vi "Mediciones4.vi"(0 "OK Button":bool, 1 "Alto":dbl, 2 "Ancho":dbl) -> ()   [LabVIEW 2017]
panel:
  out "Array":dbl[](array[numeric])
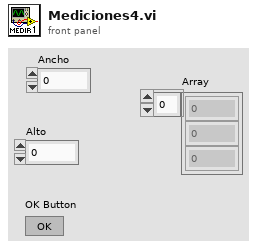
[diagram p1: front panel]
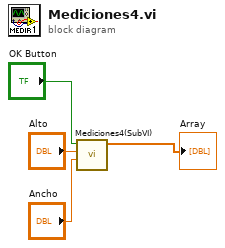
[diagram p0: block diagram]
diagram:
  n1 = call "Mediciones4(SubVI).vi"("Ancho"="Ancho", "Alto"="Alto", "OK Button"="OK Button") -> ("Array"=→"Array":dbl[])  [unwired: 8 in]
